vi "C3 to C4.vi"(8 "Command Info In":T2, 10 "C3 to C4":T1={"Target Angle"=90.0, "Distance"=45.31, "Speed"=0.75}, 11 "Starting Position":T5) -> (0 "Command Info Out":T2)   [LabVIEW 2017]
uses:
  Support Code/Starting Position.ctl
  <vilib>/Rock Robotics/WPI/Framework/Command Status Info.ctl
  <vilib>/Rock Robotics/WPI/Framework/Completion Status.ctl
  <vilib>/Rock Robotics/WPI/Framework/Completion Notifier.ctl
  Block Clusters/C3 to C4.ctl
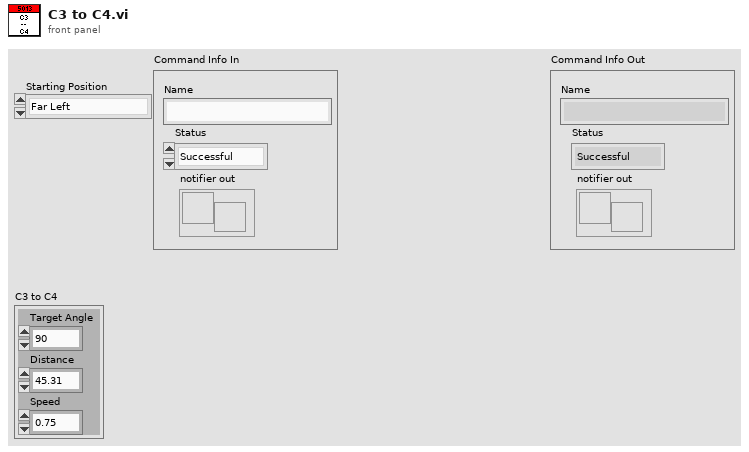
[diagram p1: front panel]
types:
  T1 = typedef "C3 to C4.ctl" = cluster{"Target Angle":dbl, "Distance":dbl, "Speed":dbl}
  T2 = typedef "Command Status Info.ctl" = cluster{"Name":string, "Status":T3, "notifier out":T4}
  T3 = typedef "Completion Status.ctl" = enum16{"Successful", "Aborted", "Incomplete"}
  T4 = typedef "Completion Notifier.ctl" = refnum<notifier>
  T5 = typedef "Starting Position.ctl" = enum16{"Far Left", "Center", "Far Right"}
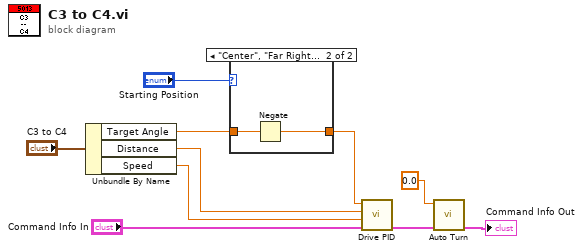
[diagram p0: block diagram]
diagram:
  n1 = Unbundle By Name("C3 to C4") -> ("Target Angle"=w3:dbl, "Distance"=w2:dbl, "Speed"=w1:dbl)
  n2 = case shown="\"Center\", \"Far Right\"" "Starting Position" {
    tunnel: [w11 w13] -> w8
    tunnel: w3 -> [w11 w12]
    frame "Far Left", Default {
    }
    frame "Center", "Far Right" {
      n3 = Negate(x=w12) -> (-x=w13:dbl)
    }
  }
  n4 = call "Drive PID.vi"("Command Info In"="Command Info In", "Speed"=w1, "Distance"=w2, "Target Angle"=w8) -> ("Command Info Out"=w10:T2)  [unwired: 7 in]
  n5 = call "Auto Turn.vi"("Command Info In"=w10, "Target Angle"=0.0) -> ("Command Info Out"=→"Command Info Out":T2)  [unwired: 9 in]
